vi "zmq unbind.vi"(8 "error in (no error)":errorcluster, 10 "addr_":string, 11 "s_":u32) -> (0 "error out":errorcluster, 2 "function return":i32, 3 "s_ out":u32)   [LabVIEW 2025, in "libzmq-v143-mt-4_3_6.lvlib"]
doc: "ZMQ_EXPORT int zmq_unbind (void *s_, const char *addr_);"
uses:
  libzmq-v143-mt-4_3_6.lvlib
  LV/LibZMQ/libzmq/lv_x86/bin/Release/libzmq-v143-mt-4_3_6.dll
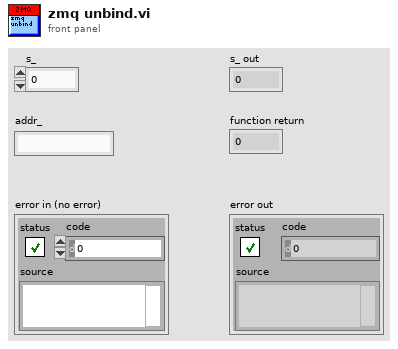
[diagram p1: front panel]
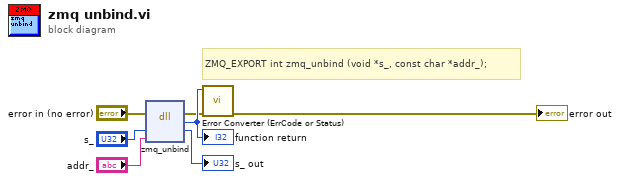
[diagram p0: block diagram]
diagram:
  # "ZMQ_EXPORT int zmq_unbind (void *s_, const char *addr_);"
  n1 = dll-call lib="C:/LV/LibZMQ/libzmq/lv_x86/bin/Release/libzmq-v143-mt-4_3_6.*" fn="zmq_unbind"(error in="error in (no error)", "s_"="s_", "addr_"="addr_") -> (error out=w2:errorcluster, w7:i32, "s_"=→"s_ out":u32)  [unwired: 3 in, 1 out]
  "function return" <- w7
  n2 = call "Error Converter (ErrCode or Status).vi"("error in (no error)"=w2, "error code"=w7) -> ("error out"=→"error out":errorcluster)  [unwired: 9 in]
